vi "ErrCheck_ROI Present.vi"(8 "Error In":errorcluster, 11 "Settings ArrayIN":T1[](array[typedef])) -> (0 "Error Out":errorcluster, 2 "Error/Warning Message":string, 3 "ROI Descriptor Missing?":bool)   [LabVIEW 2012]
doc: "SciScan 1.2 160622"
uses:
  MacroGUI Module/Custom Controls and Typedefs/GFG Variable for IO.ctl
  GFG/GFG library.lvlib
  GFG/GFGnumericGet.vi
  GFG/GFGbooleanGet.vi
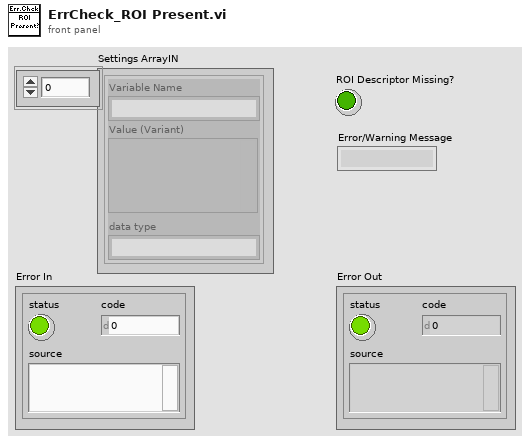
[diagram p1: front panel]
types:
  T1 = typedef "GFG Variable for IO.ctl" = cluster{"Variable Name":string, "Value (Variant)":variant, "data type":string}
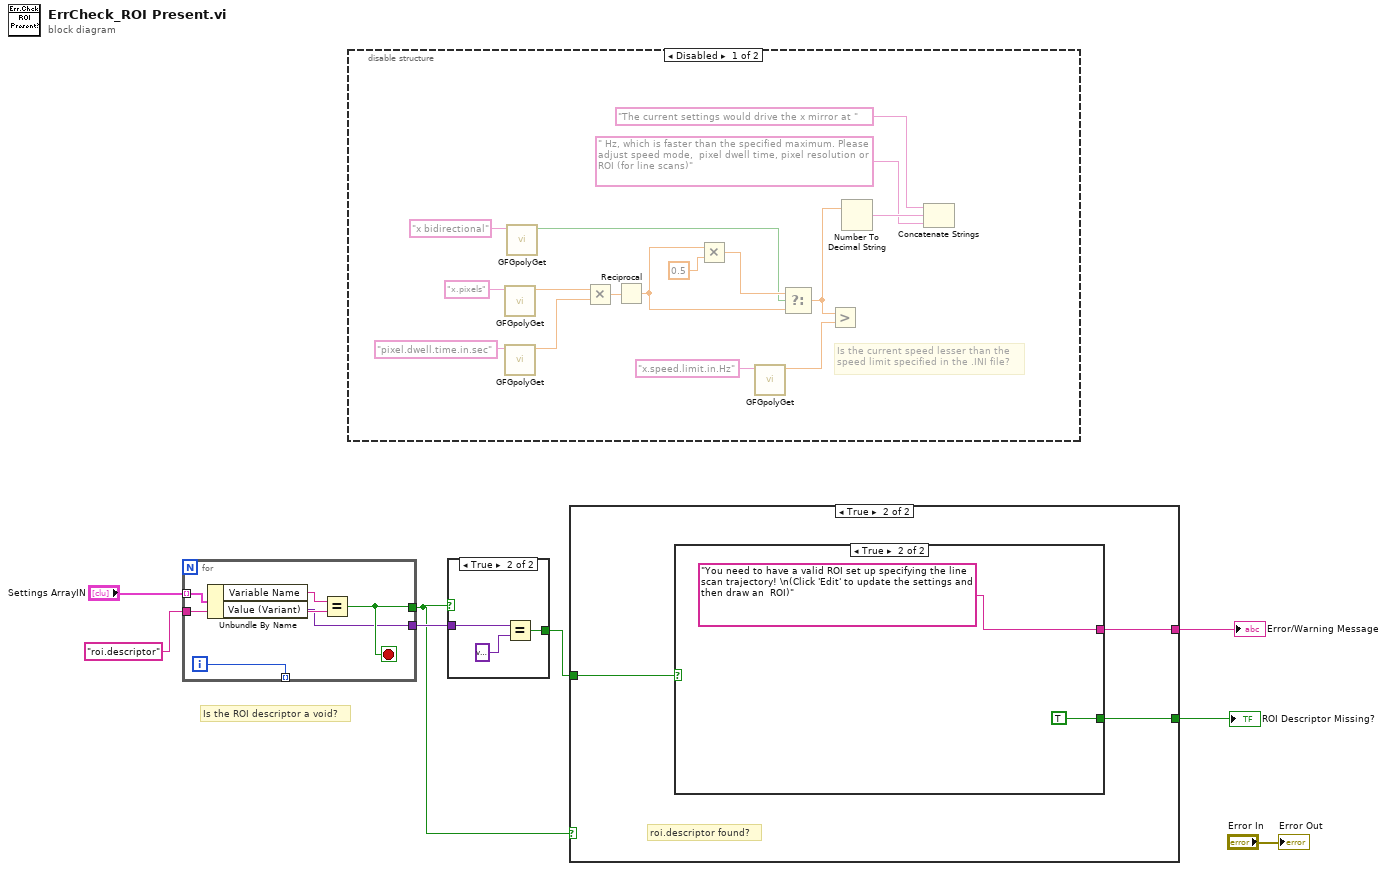
[diagram p0: block diagram]
diagram:
  # "Is the ROI descriptor a void?"
  n1 = for {
    tunnel: "Settings ArrayIN" -> [w14] mode=indexing
    tunnel: "roi.descriptor" ("Variable Name in") -> [w12]
    tunnel: [w11] -> w2
    tunnel: [w10] -> _ mode=indexing
    tunnel: [w9] -> w3
    i -> [w10]
    stop <- w11 stop-if-true
    n2 = Unbundle By Name(w14) -> ("Variable Name"=w13:string, "Value (Variant)"=w9:variant)
    n3 = Equal?(x=w13, y=w12) -> (x = y?=w11:bool)
  }
  n4 = disable-structure shown="Disabled" {
    frame Disabled {
      # "Is the current speed lesser than the\nspeed limit specified in the .INI file?"
      n5 = call-poly "GFGpolyGet.vi"("Variable Name in"="x.pixels") -> ("Numeric"=w20:dbl)  [unwired: 8 in, 2 out]
      n6 = call-poly "GFGpolyGet.vi"("Variable Name in"="pixel.dwell.time.in.sec") -> ("Numeric"=w19:dbl)  [unwired: 8 in, 2 out]
      n7 = call-poly "GFGpolyGet.vi"("Variable Name in"="x bidirectional") -> ("Boolean Value OUT"=w21:bool)  [unwired: 9 in, 1 out]
      n8 = Multiply(x=w20, y=w19) -> (x*y=w22:dbl)
      n9 = Reciprocal(x=w22) -> (1/x=w23:dbl)
      n10 = Multiply(x=w23, y=0.5) -> (x*y=w24:dbl)
      n11 = call-poly "GFGpolyGet.vi"("Variable Name in"="x.speed.limit.in.Hz") -> ("Numeric"=w27:dbl)  [unwired: 8 in, 2 out]
      n12 = Select(t=w24, s=w21, f=w23) -> (s? t:f=w15:dbl)
      n13 = Greater?(x=w15, y=w27) -> ()  [unwired: 1 out]
      n14 = Number To Decimal String(number=w15) -> (decimal integer string=w17:string)  [unwired: 1 in]
      n15 = Concatenate Strings("The current settings would drive the x mirror at " ("message"), w17, " Hz, which is faster than the specified maximum. Please adjust speed mode,  pixel dwell time, pixel resolution or ROI (for line scans)" ("string")) -> ()  [unwired: 1 out]
    }
    frame Enabled {
    }
  }
  n16 = case shown="True" w2 {
    tunnel: w3 -> [_ w32]
    tunnel: [_ w31] -> w1
    frame False {
    }
    frame True {
      n17 = Equal?(x=w32, y=variant) -> (x = y?=w31:bool)
    }
  }
  n18 = case shown="True" w2 {
    tunnel: [_ w35] -> w7
    tunnel: w1 -> [_ w36]
    tunnel: [_ w34] -> w6
    frame False {
      # "Donot run the speed check for RESO system"
    }
    frame True {
      # "roi.descriptor found?"
      n19 = case shown="True" w36 {
        tunnel: [_ TRUE] -> w35
        tunnel: [_ "You need to have a valid ROI set up specifying the line scan trajectory! \n(Click 'Edit' to update the settings and then draw an  ROI)" ("string")] -> w34
        frame False {
        }
        frame True {
        }
      }
    }
  }
  "ROI Descriptor Missing?" <- w7
  "Error/Warning Message" <- w6
  "Error Out" <- "Error In"
